vi "extrinsic_matrix.vi"(10 "corner":dbl[][](array[numeric])) -> (3 "extrinsic":dbl[][](array[numeric]))   [LabVIEW 2017]
panel:
  out "x/y":dbl
  out "floor(x/y)":dbl
  out "Numeric":dbl
  out "X":dbl[][](array[numeric])
  out "X'":dbl[][](array[numeric])
  out "angle":dbl
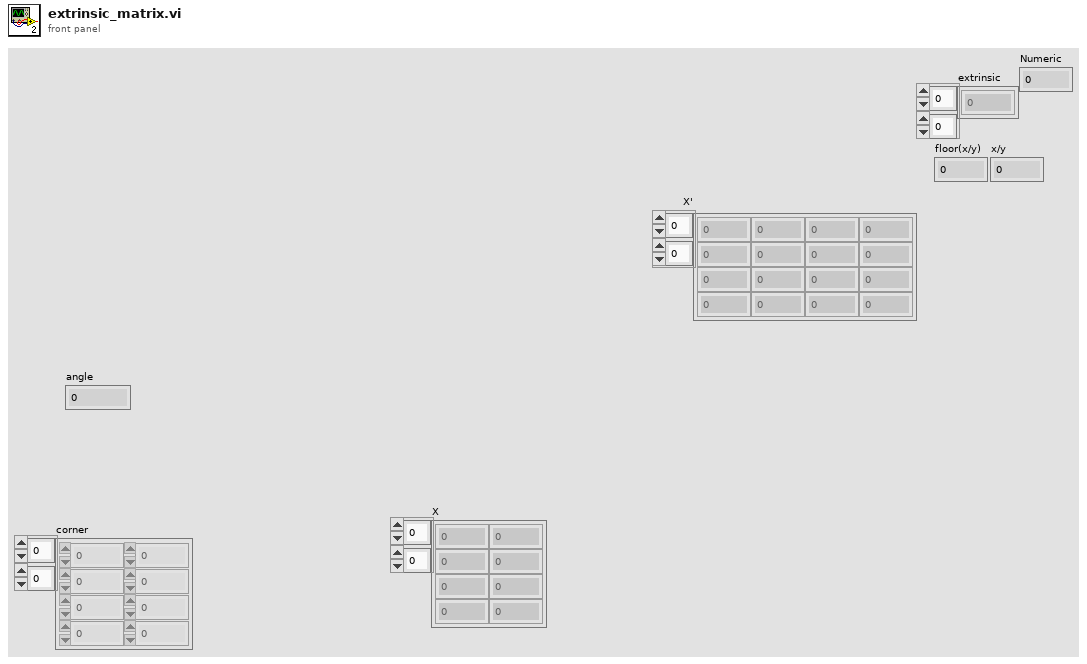
[diagram p1: front panel]
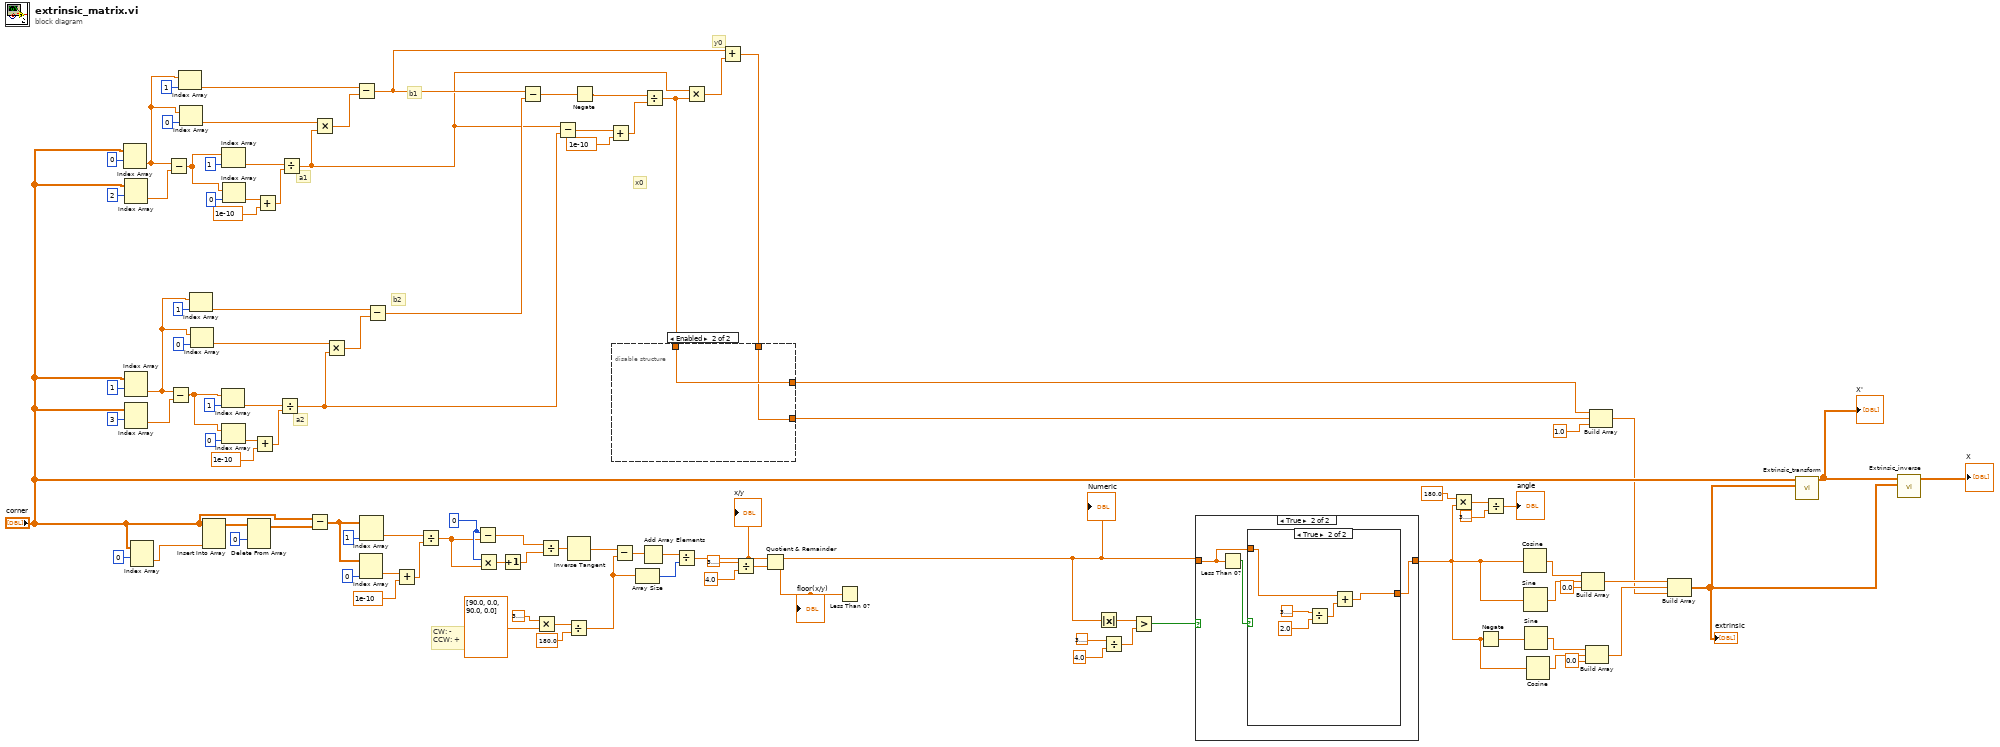
[diagram p0: block diagram]
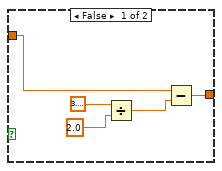
[diagram p3: hidden frame]
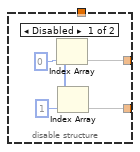
[diagram p4: hidden frame]
diagram:
  w88 = 0
  # "y0"
  # "x0"
  # "a2"
  # "b2"
  # "a1"
  # "b1"
  # "CW: -\nCCW: +"
  n1 = Index Array(array="corner", index (row)=0) -> (element=w54:dbl[])  [unwired: 1 in]
  n2 = Index Array(array="corner", index (row)=2) -> (element=w66:dbl[])  [unwired: 1 in]
  n3 = Index Array(array="corner", index (row)=1) -> (element=w49:dbl[])  [unwired: 1 in]
  n4 = Index Array(array="corner", index (row)=3) -> (element=w65:dbl[])  [unwired: 1 in]
  n5 = Index Array(array="corner", index (row)=0) -> (element=w103:dbl[])  [unwired: 1 in]
  n6 = Subtract(x=w54, y=w66) -> (x-y=w62:dbl[])
  n7 = Subtract(x=w49, y=w65) -> (x-y=w57:dbl[])
  n8 = Index Array(array=w54, index=1 ("index (row)")) -> (element=w53:dbl)
  n9 = Index Array(array=w54, index=0 ("index (row)")) -> (element=w44:dbl)
  n10 = Index Array(array=w49, index=1 ("index (row)")) -> (element=w50:dbl)
  n11 = Index Array(array=w49, index=0 ("index (row)")) -> (element=w43:dbl)
  n12 = Insert Into Array(array="corner", new element=w103) -> (w102:dbl[][])  [unwired: 2 in]
  n13 = Index Array(array=w57, index=1 ("index (row)")) -> (element=w60:dbl)
  n14 = Index Array(array=w62, index=1 ("index (row)")) -> (element=w61:dbl)
  n15 = Index Array(array=w57, index=0 ("index (row)")) -> (element=w19:dbl)
  n16 = Index Array(array=w62, index=0 ("index (row)")) -> (element=w21:dbl)
  n17 = Delete From Array(array=w102, index (row)=0 ("length")) -> (array with subset deleted=w100:dbl[][])  [unwired: 2 in, 1 out]
  n18 = Add(x=w19, y=1e-10) -> (x+y=w18:dbl)
  n19 = Add(x=w21, y=1e-10) -> (x+y=w20:dbl)
  n20 = Divide(x=w60, y=w18) -> (x/y=w45:dbl)
  n21 = Divide(x=w61, y=w20) -> (x/y=w40:dbl)
  n22 = Subtract(x="corner", y=w100) -> (x-y=w97:dbl[][])
  n23 = Multiply(x=w44, y=w40) -> (x*y=w47:dbl)
  n24 = Multiply(x=w43, y=w45) -> (x*y=w46:dbl)
  n25 = Subtract(x=w53, y=w47) -> (x-y=w41:dbl)
  n26 = Index Array(array=w97, index (col)=0 ("disabled index (col)")) -> (element=w26:dbl[])  [unwired: 1 in]
  n27 = Index Array(array=w97, index (col)=1 ("disabled index (col)")) -> (element=w96:dbl[])  [unwired: 1 in]
  n28 = Subtract(x=w50, y=w46) -> (x-y=w48:dbl)
  n29 = Add(x=w26, y=1e-10) -> (x+y=w25:dbl[])
  n30 = Divide(x=w96, y=w25) -> (x/y=w85:dbl[])
  n31 = Subtract(x=w88, y=w85) -> (x-y=w95:dbl[])
  n32 = Multiply(x=w88, y=w85) -> (x*y=w89:dbl[])
  n33 = Increment(x=w89) -> (x+1=w90:dbl[])
  n34 = Subtract(x=w41, y=w48) -> (x-y=w37:dbl)
  n35 = Multiply(x=3.141592653589793, y=dbl[] [90.0, 0.0, 90.0, 0.0] ("x/y")) -> (x*y=w84:dbl[])
  n36 = Divide(x=w95, y=w90) -> (x/y=w91:dbl[])
  n37 = Subtract(x=w40, y=w45) -> (x-y=w16:dbl)
  n38 = Divide(x=w84, y=180.0 ("x")) -> (x/y=w78:dbl[])
  n39 = Inverse Tangent(1:w91) -> (0:w80:dbl[])
  n40 = Negate(x=w37) -> (-x=w38:dbl)
  n41 = Add(x=w16, y=1e-10) -> (x+y=w15:dbl)
  n42 = Subtract(x=w80, y=w78) -> (x-y=w79:dbl[])
  n43 = Array Size(array=w78) -> (size(s)=w86:i32)
  n44 = Add Array Elements(numeric array=w79) -> (sum=w87:dbl)
  n45 = Divide(x=w38, y=w15) -> (x/y=w28:dbl)
  n46 = Divide(x=w87, y=w86) -> (x/y=w3:dbl)
  "x/y" <- w3
  n47 = Multiply(x=w40, y=w28) -> (x*y=w42:dbl)
  n48 = Add(x=w41, y=w42) -> (x+y=w27:dbl)
  n49 = disable-structure shown="Enabled" {
    disable-tunnel: [w106 w111] -> w31
    disable-tunnel: [w105 w110] -> w30
    disable-tunnel: w28 -> [_ w111]
    disable-tunnel: w27 -> [_ w110]
    frame Disabled {
      n50 = Index Array(index=0 ("index (row)")) -> (array=w107:i32[], element=w106)
      n51 = Index Array(array=w107, index=1 ("index (row)")) -> (element=w105)
    }
    frame Enabled {
    }
  }
  n52 = Divide(x=3.141592653589793, y=4.0) -> (x/y=w12:dbl)
  n53 = Quotient & Remainder(x=w3, y=w12) -> (x-y*floor(x/y)=w1:dbl, floor(x/y)=w11:dbl)
  "Numeric" <- w1
  "floor(x/y)" <- w11
  n54 = Less Than 0?(x=w11) -> ()  [unwired: 1 out]
  n55 = Absolute Value(x=w1) -> (abs(x)=w8:dbl)
  n56 = Divide(x=3.141592653589793, y=4.0) -> (x/y=w7:dbl)
  n57 = Greater?(x=w8, y=w7) -> (0:w6:bool)
  n58 = case shown="True" w6 {
    tunnel: w1 -> [w112 w114]
    tunnel: [w112 w113] -> w2
    frame False {
    }
    frame True {
      n59 = Less Than 0?(x=w114) -> (x < 0?=w115:bool)
      n60 = case shown="True" w115 {
        tunnel: w114 -> [w116 w122]
        tunnel: [w118 w121] -> w113
        frame False {
          n61 = Divide(x=3.141592653589793, y=2.0) -> (x/y=w117:dbl)
          n62 = Subtract(x=w116, y=w117) -> (x-y=w118:dbl)
        }
        frame True {
          n63 = Divide(x=3.141592653589793, y=2.0) -> (x/y=w123:dbl)
          n64 = Add(x=w122, y=w123) -> (x+y=w121:dbl)
        }
      }
    }
  }
  n65 = Multiply(x=180.0, y=w2) -> (x*y=w94:dbl)
  n66 = Negate(x=w2) -> (-x=w39:dbl)
  n67 = Divide(x=w94, y=3.141592653589793) -> (x/y=→"angle":dbl)
  n68 = Cosine(x=w2) -> (cos(x)=w76:dbl)
  n69 = Sine(x=w2) -> (sin(x)=w75:dbl)
  n70 = Sine(x=w39) -> (sin(x)=w74:dbl)
  n71 = Cosine(x=w2) -> (cos(x)=w73:dbl)
  n72 = Build Array(w76, w75, 0.0 ("element")) -> (w72:dbl[])
  n73 = Build Array(w74, w73, 0.0 ("element")) -> (w71:dbl[])
  n74 = Build Array(w31, w30, 1.0 ("element")) -> (w32:dbl[])
  n75 = Build Array(w72, w71, w32) -> (w29:dbl[][])
  "extrinsic" <- w29
  n76 = call "Extrinsic_transform.vi"("extrinsic"=w29, "X"="corner") -> ("X'"=w5:dbl[][])  [unwired: 9 in]
  "X'" <- w5
  n77 = call "Extrinsic_inverse.vi"("extrinsic"=w29, "X'"=w5) -> ("X'"=→"X":dbl[][])  [unwired: 9 in]
